vi "Volt and Trigger1.vi"() -> ()   [LabVIEW 2014]
uses:
  <vilib>/Utility/error.llb/DialogType.ctl
  <vilib>/_DAQmxBase/Internals/DAQmxBase Create Channel (AI-Voltage-Basic).vi
  <vilib>/_DAQmxBase/Internals/DAQmxBase Timing (Sample Clock).vi
  <vilib>/_DAQmxBase/Internals/DAQmxBase Read (Analog 2D DBL NChan NSamp).vi
panel:
  out "Pre-Trigger Error":bool caption="Error \n(Triggered before\n pretrigger samples\n were acquired)"
  in  "Samples to Read":i32 caption="Index of Condition Channel"
  in  "Pretrigger Samples":i32
  in  "Index of Condition Channel":i32
  in  "Level":sgl
  in  "Window Amplitude":sgl step=0.1 format="%0.2f"
  in  "Condition":T1(ring)
  in  "units":i32(ring)=10348 items=["Volts"=10348, "From Custom Scale"=10065]
  in  "stop":bool
  out "Waveform Chart":dbl[][](graph)
  in  "physical channels":tag
  in  "maximum value":dbl=5.0 format="%0.2f"
  in  "minimum value":dbl=-5.0 format="%0.2f"
  in  "rate":i32=1000 caption="Sample Rate"
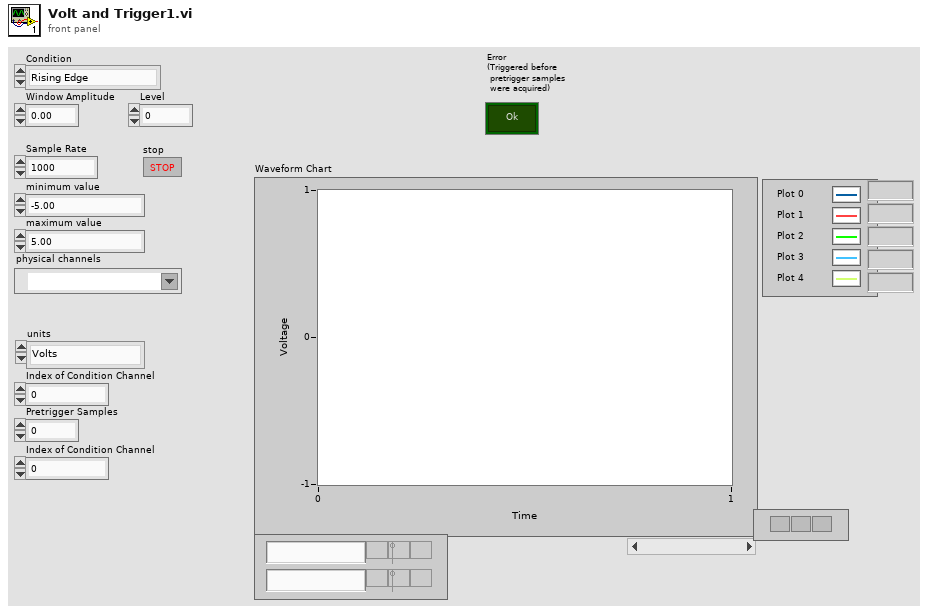
[diagram p1: front panel]
types:
  T1 = enum16{"Rising Edge", "Falling Edge", "Above Level", "Below Level", "When Inside Window", "When Outside Window"}
  T2 = typedef "DialogType.ctl" = u16
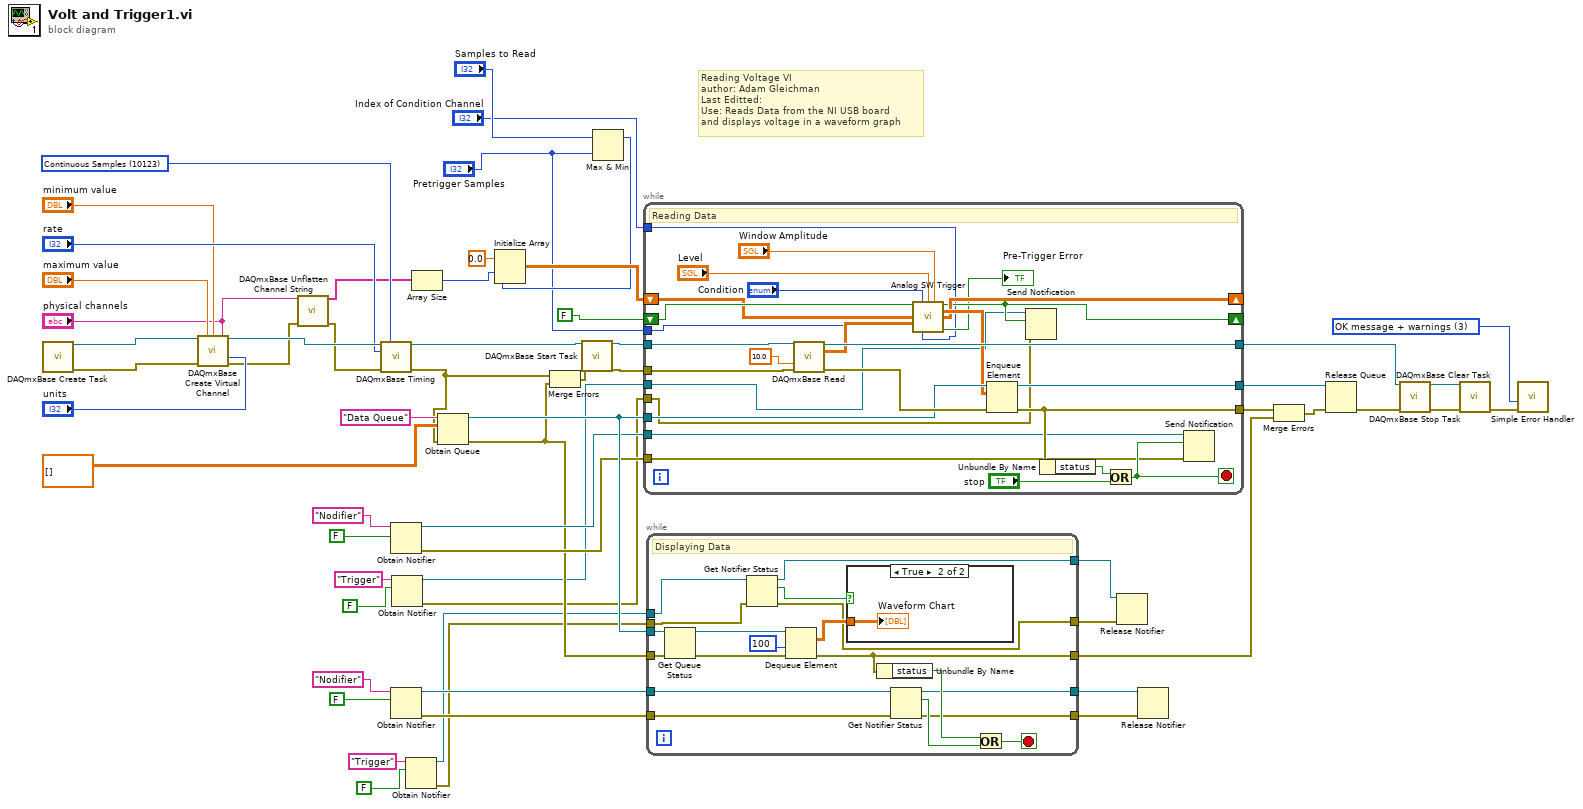
[diagram p0: block diagram]
diagram:
  w40 = 10123 items=["Finite Samples"=10178, "Continuous Samples"=10123, "Hardware Timed Single Point"=12522] ("sample mode")
  w42 = T2 3 items=["no dialog", "OK message", "continue or stop message", "OK message + warnings", "continue/stop + warnings"] ("type of dialog (OK msg:1)")
  # "Reading Voltage VI\nauthor: Adam Gleichman\nLast Editted: \nUse: Reads Data from the NI USB board\nand displays voltage in a waveform graph"
  n1 = call <vilib>:"DAQmxBase Create Task.vi"() -> ("task out"=w58:refnum<k21>, "error out"=w57:errorcluster)  [unwired: 5 in, 9 out]
  n2 = call-poly <vilib>:"DAQmxBase Create Virtual Channel.vi"("task in"=w58, "maximum value"="maximum value", "minimum value"="minimum value", "physical channels"="physical channels", "units"="units", "error in"=w57) -> ("task out"=w56:refnum<k21>, "error out"=w21:errorcluster)  [unwired: 3 in, 5 out]
  n3 = call "DAQmxBase Unflatten Channel String.vi"("names in"="physical channels", "error in"=w21) -> ("names out"=w18:string[], "error out"=w20:errorcluster)  [unwired: 12 in]
  n4 = call-poly <vilib>:"DAQmxBase Timing.vi"("task/channels in"=w56, "sample mode"=w40, "rate"="rate", "error in"=w20) -> ("task out"=w27:refnum<k21>, "error out"=w26:errorcluster)  [unwired: 3 in, 7 out]
  n5 = Obtain Notifier(name (unnamed)="Nodifier", notification data type=FALSE) -> (notifier out=w36:refnum<notifier>, error out=w35:errorcluster)  [unwired: 2 in, 1 out]
  n6 = Obtain Notifier(name (unnamed)="Nodifier", notification data type=FALSE) -> (notifier out=w33:refnum<notifier>, error out=w31:errorcluster)  [unwired: 2 in, 1 out]
  n7 = Obtain Notifier(name (unnamed)="Trigger", notification data type=FALSE) -> (notifier out=w9:refnum<notifier>, error out=w8:errorcluster)  [unwired: 2 in, 1 out]
  n8 = Obtain Notifier(name (unnamed)="Trigger", notification data type=FALSE) -> (notifier out=w5:refnum<notifier>, error out=w4:errorcluster)  [unwired: 2 in, 1 out]
  n9 = Array Size(array=w18) -> (size(s)=w17:i32)
  n10 = Obtain Queue(name (unnamed)="Data Queue", element data type=dbl[][] [] ("data"), error in (no error)=w26) -> (queue out=w48:refnum<queue>, error out=w25:errorcluster)  [unwired: 2 in, 1 out]
  n11 = Merge Errors(w26, w25) -> (w28:errorcluster)
  n12 = call <vilib>:"DAQmxBase Start Task.vi"("task/channels in"=w27, "error in"=w28) -> ("task out"=w24:refnum<k21>, "error out"=w23:errorcluster)  [unwired: 12 out]
  n13 = Max & Min(x="Samples to Read", y="Pretrigger Samples") -> (max(x,y)=w13:i32)  [unwired: 1 out]
  n14 = Initialize Array(0.0 ("element"), w17, w13) -> (w15:dbl[][])
  n15 = while "Data Reading Loop" {
    tunnel: w48 -> [w85]
    tunnel: [w83] -> w51
    tunnel: [w81] -> w50
    tunnel: [w79] -> w39
    tunnel: w36 -> [w77]
    tunnel: w35 -> [w76]
    tunnel: w24 -> [w75]
    tunnel: w23 -> [w74]
    shift-right: [w65] -> _
    shift-left: w15 -> [w67]
    shift-right: [w64] -> _
    shift-left: FALSE -> [w68]
    tunnel: "Pretrigger Samples" -> [w66]
    tunnel: w9 -> [w63]
    tunnel: w8 -> [w62]
    tunnel: "Index of Condition Channel" -> [w60]
    stop <- w78 stop-if-true
    # "Reading Data"
    n16 = call-poly <vilib>:"DAQmxBase Read.vi"("task/channels in"=w75, "timeout"=10.0, "error in"=w74) -> ("task out"=w79:refnum<k21>, "data"=w73:dbl[][], "error out"=w86:errorcluster)  [unwired: 10 in]
    n17 = call "Analog SW Trigger.vi"("Triggered?"=w68, "Condition"="Condition", "Level"="Level", "Window Amplitude"="Window Amplitude", "Initialized Data Array"=w67, "Input Raw Data"=w73, "Pretrigger Samples"=w66, "Index of Condition Channel"=w60) -> ("Trigger Out"=w64:bool, "Output Data (Scaled)"=w72:dbl[][], "Raw Data Out"=w65:dbl[][], "Pre-Trigger Error"=→"Pre-Trigger Error":bool)  [unwired: 3 in, 1 out]
    n18 = Enqueue Element(queue=w85, element=w72, error in (no error)=w86) -> (queue out=w83:refnum<queue>, error out=w81:errorcluster)  [unwired: 1 in, 1 out]
    n19 = Send Notification(notification=w64, notifier=w63, error in (no error)=w62) -> ()  [unwired: 2 out]
    n20 = Unbundle By Name(w81) -> ("status"=w80:bool)
    n21 = Or(x=w80, y="stop") -> (x .or. y?=w78:bool)
    n22 = Send Notification(notification=w78, notifier=w77, error in (no error)=w76) -> ()  [unwired: 2 out]
  }
  n23 = while {
    tunnel: w48 -> [w105]
    tunnel: w25 -> [w93]
    tunnel: [w103] -> w47
    tunnel: w33 -> [w100]
    tunnel: w31 -> [w99]
    tunnel: [w97] -> w29
    tunnel: [w96] -> w30
    tunnel: w5 -> [w91]
    tunnel: w4 -> [w90]
    tunnel: [w88] -> w3
    tunnel: [w87] -> w2
    stop <- w101 stop-if-true
    # "Displaying Data"
    n24 = Get Queue Status(queue=w105, error in (no error)=w93) -> (queue out=w94:refnum<queue>, error out=w92:errorcluster)  [unwired: 1 in, 6 out]
    n25 = Get Notifier Status(notifier=w91, error in (no error)=w90) -> (notifier out=w88:refnum<notifier>, current notification=w89:bool, error out=w87:errorcluster)  [unwired: 2 out]
    n26 = Dequeue Element(queue=w94, timeout in ms (-1)=100, error in (no error)=w92) -> (element=w95:dbl[][], error out=w103:errorcluster)  [unwired: 2 out]
    n27 = case shown="True" w89 {
      tunnel: w95 -> [_ w106]
      frame False {
      }
      frame True {
        "Waveform Chart" <- w106
      }
    }
    n28 = Unbundle By Name(w103) -> ("status"=w102:bool)
    n29 = Get Notifier Status(notifier=w100, error in (no error)=w99) -> (notifier out=w97:refnum<notifier>, current notification=w98:bool, error out=w96:errorcluster)  [unwired: 2 out]
    n30 = Or(x=w102, y=w98) -> (x .or. y?=w101:bool)
  }
  n31 = Release Notifier(notifier=w3, error in (no error)=w2) -> ()  [unwired: 1 in, 3 out]
  n32 = Release Notifier(notifier=w29, error in (no error)=w30) -> ()  [unwired: 1 in, 3 out]
  n33 = Merge Errors(w50, w47) -> (w49:errorcluster)
  n34 = Release Queue(queue=w51, error in (no error)=w49) -> (error out=w46:errorcluster)  [unwired: 1 in, 2 out]
  n35 = call <vilib>:"DAQmxBase Stop Task.vi"("task/channels in"=w39, "error in"=w46) -> ("task out"=w45:refnum<k21>, "error out"=w44:errorcluster)  [unwired: 12 in]
  n36 = call <vilib>:"DAQmxBase Clear Task.vi"("task in"=w45, "error in"=w44) -> ("error out"=w43:errorcluster)  [unwired: 13 in]
  n37 = call <vilib>:"Simple Error Handler.vi"("type of dialog (OK msg:1)"=w42, "error in (no error)"=w43) -> ()  [unwired: 3 in, 5 out]
